vi "Configure Acquisition.vi"(8 "error in (no error)":errorcluster, 9 "Number of Waveform Acquisitions (16)":i32=16, 10 "Acquisition Type (0: Sample)":u16(ring) items=["Sample", "Peak Detect", "Hi Res", "Envelope", "Average"], 11 "VISA resource name":refnum<visa-resource-name>) -> (0 "error out":errorcluster, 3 "VISA resource name out":refnum<visa-resource-name>)   [LabVIEW 2016, in "Tektronix DPO MSO 2000 4000 Series.lvlib"]
doc: "Configures the acquisition method for the oscilloscope."
uses:
  Tektronix DPO MSO 2000 4000 Series.lvlib
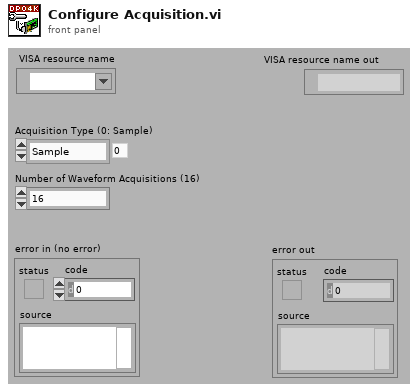
[diagram p1: front panel]
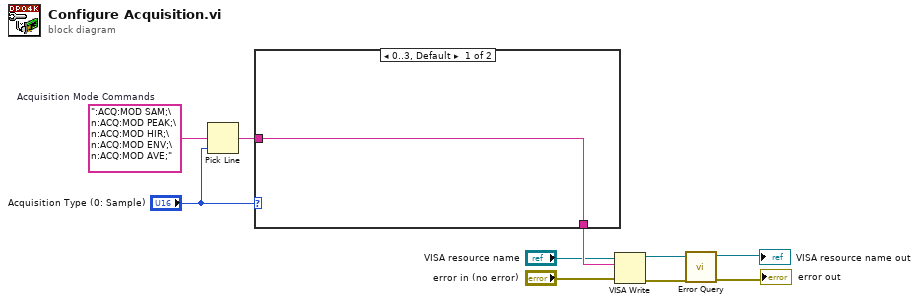
[diagram p0: block diagram]
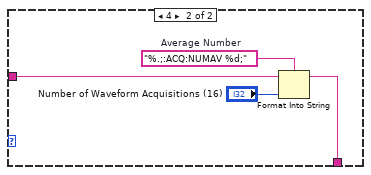
[diagram p2: hidden frame]
diagram:
  w10 = ":ACQ:MOD SAM;\n:ACQ:MOD PEAK;\n:ACQ:MOD HIR;\n:ACQ:MOD ENV;\n:ACQ:MOD AVE;"  # Acquisition Mode Commands
  n1 = Pick Line(multi-line string=w10, line index="Acquisition Type (0: Sample)") -> (output string=w8:string)  [unwired: 1 in]
  n2 = case shown="0..3, Default" "Acquisition Type (0: Sample)" {
    tunnel: w8 -> [w11 w15]
    tunnel: [w11 w12] -> w7
    frame 0..3, Default {
    }
    frame 4 {
      w14 = "%.;:ACQ:NUMAV %d;"  # Average Number
      n3 = Format Into String(format string=w14, initial string=w15, "Number of Waveform Acquisitions (16)") -> (resulting string=w12:string)  [unwired: 1 in, 1 out]
    }
  }
  n4 = VISA Write(VISA resource name="VISA resource name", write buffer=w7, error in (no error)="error in (no error)") -> (VISA resource name out=w4:refnum<visa-resource-name>, error out=w3:errorcluster)  [unwired: 1 out]
  n5 = call "Error Query.vi"("error in (no error)"=w3, "VISA resource name"=w4) -> ("error out"=→"error out":errorcluster, "VISA resource name out"=→"VISA resource name out":refnum<visa-resource-name>)  [unwired: 6 in, 2 out]
